vi "Unregister (async).vi"(7 "Options":string, 8 "error in (no error)":errorcluster, 10 "Endpoint URI":string, 11 "WAMP Client in":refnum<class "WAMP Client.lvclass">) -> (0 "error out":errorcluster, 2 "notifier out":refnum<notifier>, 3 "WAMP Client out":refnum<class "WAMP Client.lvclass">)   [LabVIEW 2020, in "wamplv.lvlib" / "WAMP Client.lvclass"]
uses:
  WAMP Client.lvclass
  TypeDef/Success or error.ctl
  API/TypeDefs/Combined error.ctl
  API/TypeDefs/WAMP error.ctl
  TypeDef/Internal Message Type.ctl
  TypeDef/Unregister request.ctl
  WAMP Client.lvclass/WAMP Client.ctl
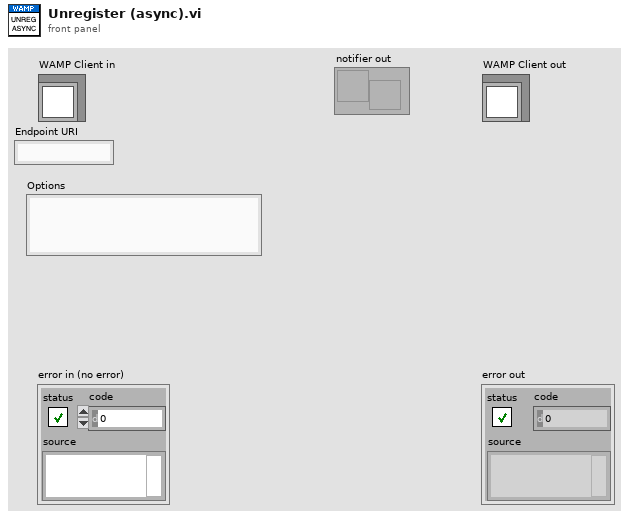
[diagram p1: front panel]
types:
  T1 = typedef "wamplv.lvlib/WAMP Client.lvclass/Unregister request.ctl" = cluster{"URI":string, "Unregister result notifier":refnum<notifier>, "Options":string}
  T2 = typedef "wamplv.lvlib/WAMP Client.lvclass/Success or error.ctl" = cluster{"Success?":bool, "URI":string, "Combined Error":T3}
  T3 = typedef "wamplv.lvlib/WAMP Client.lvclass/Combined error.ctl" = cluster{"Error?":bool, "WAMP Error":T4, "Error":errorcluster}
  T4 = typedef "wamplv.lvlib/WAMP Client.lvclass/WAMP error.ctl" = cluster{"Details":string, "ArgumentKw Payload":string, "Error?":bool, "Error URI":string, "Arguments Payload":string}
  T5 = typedef "wamplv.lvlib/WAMP Client.lvclass/Internal Message Type.ctl" = enum16{"Subscribe", "Handle Subscribed", "Handle Event", "Unsubscribe", "Handle Unsubscribed", "Publish", "Handled Published", "Goodbye", "Handle Goodbye", "Call", "Handle Result", "Register", "Handle Registered", "Unregister", "Handle Unregistered", "Handle Invocation", "Yield", "Error"}
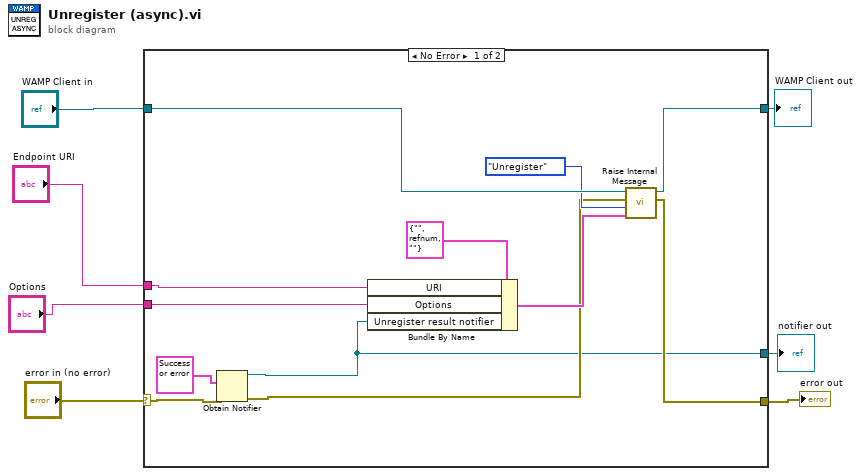
[diagram p0: block diagram]
diagram:
  n1 = case shown="No Error" "error in (no error)" {
    selector: "error in (no error)" -> [w13 w21]
    tunnel: [w15 w21] -> w6
    tunnel: [w14 w20] -> w4
    tunnel: "WAMP Client in" -> [w19 w20]
    tunnel: [w11 _] -> w2
    tunnel: "Endpoint URI" -> [w9 _]
    tunnel: "Options" -> [w8 _]
    frame No Error {
      n2 = Obtain Notifier(notification data type=T2 {"Success?"=FALSE, "URI"="", "Combined Error"={"Error?"=FALSE, "WAMP Error"={"Details"="{}", "ArgumentKw Payload"="{}", "Error?"=FALSE, "Error URI"="", "Arguments Payload"=""}, "Error"={"status"=FALSE, "code"=0, "source"=""}}} ("Sucess or error"), error in (no error)=w13) -> (notifier out=w11:refnum<notifier>, error out=w12:errorcluster)  [unwired: 2 in, 1 out]
      n3 = Bundle By Name(cluster=T1 {"URI"="", "Unregister result notifier"=refnum, "Options"=""} ("Unregister Request"), "URI"=w9, "Options"=w8, "Unregister result notifier"=w11) -> (w18:T1)
      n4 = call "Raise Internal Message.vi"("Variant"=w18, "Internal Message Type"=Internal_Message_Type."Unregister", "error in (no error)"=w12, "WAMP Client in"=w19) -> ("error out"=w15:errorcluster, "WAMP Client out"=w14:refnum<class "WAMP Client.lvclass">)  [unwired: 6 in]
    }
    frame Error {
    }
  }
  "error out" <- w6
  "WAMP Client out" <- w4
  "notifier out" <- w2
